vi "Measurement Logic.vi"(8 "error in":errorcluster, 9 "measurement configuration":T2={"Resource Name(s)"=[], "Number Of Records"=32, "Timeout (s)"=1.2, "Configuration File Path"="", "Delay Mode"="On", "Horizontal Position"=0.0, "Length Unit"="Percentage", "Record Length"=100.0, "Stream To File Path"=""} {"Record Length" format="%#_6ps"; "Horizontal Position" min=0.0 max=100.0 step=5.0 format="%#_6ps"; "Timeout (s)" format="%#_6p"}, 10 "measure call context in":refnum<class "Measure Call Context.lvclass">) -> (0 "error out":errorcluster, 1 "measurement results":T1={"RelativeInitialX"=[0.0], "xIncrement"=[0.0], "Wfm"=[[0.0]], "Plot Names"=[], "Actual Sample Rate"=10000000.0, "Actual Record Duration"=0.0, "Actual Record Length"=256.0} {"Actual Record Length" format="%#_6p Samples"; "Actual Record Duration" format="%#_6p Samples"; "Actual Sample Rate" format="%#_6ps"}, 2 "measure call context out":refnum<class "Measure Call Context.lvclass">)   [LabVIEW 2025, in "Ni-Scope-Multirecords.lvclass"]
doc: "Contains the core logic for executing the measurement."
uses:
  Ni-Scope-Multirecords.lvclass
  <vilib>/Plug-In SDKs/Measurements/Measure Call Context/Measure Call Context.lvclass
  Measurement Configuration.ctl
  Measurement Results.ctl
  <vilib>/Plug-In SDKs/Measurements/Measure Call Context/Reserve Sessions - NPin.vi
  <vilib>/Plug-In SDKs/Sessions/niScope/Initialize Sessions - 1Sess.vi
  <extravilib>/ChannelInstances/Event Messenger-bool/Instantiate.vi
  Ni-Scope-Multirecords.lvclass/Ni-Scope-Multirecords.ctl
  <vilib>/Plug-In SDKs/Sessions/niScope/NI Session Management niScope.lvlib
  <vilib>/Plug-In SDKs/Clients/Session Management V1/Session Reservation/Session Reservation.lvclass
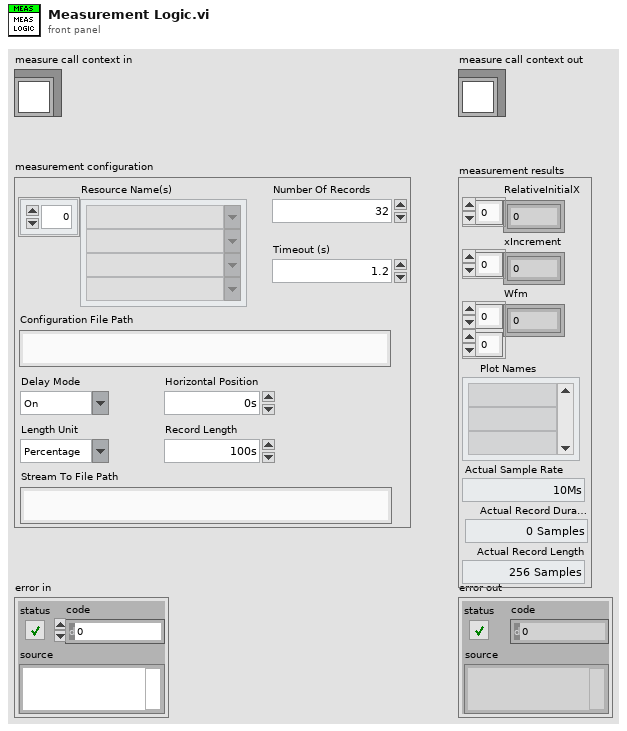
[diagram p1: front panel]
types:
  T1 = typedef "Ni-Scope-Multirecords.lvclass/Measurement Results.ctl" = cluster{"RelativeInitialX":dbl[], "xIncrement":dbl[], "Wfm":dbl[][], "Plot Names":string[], "Actual Sample Rate":dbl, "Actual Record Duration":dbl, "Actual Record Length":dbl}
  T2 = typedef "Ni-Scope-Multirecords.lvclass/Measurement Configuration.ctl" = cluster{"Resource Name(s)":string[], "Number Of Records":i32, "Timeout (s)":dbl, "Configuration File Path":string, "Delay Mode":string, "Horizontal Position":dbl, "Length Unit":string, "Record Length":dbl, "Stream To File Path":string}
  T3 = cluster{"Actual Sample Rate":dbl, "Actual Record Duration":dbl, "Actual Record Length":i32}
  T4 = typedef "Ni-Scope-Multirecords.lvclass/Recording Settings.ctl" = cluster{"Number of Records":i32, "Plot Names":string[][], "Stream To File?":bool, "TDMS Session":refnum<k34>, "Fetch Timeout":dbl, "Channels Per Record":i32}
  T5 = typedef "Event Messenger-bool.lvlib/))Channel.ctl" = refnum<queue>
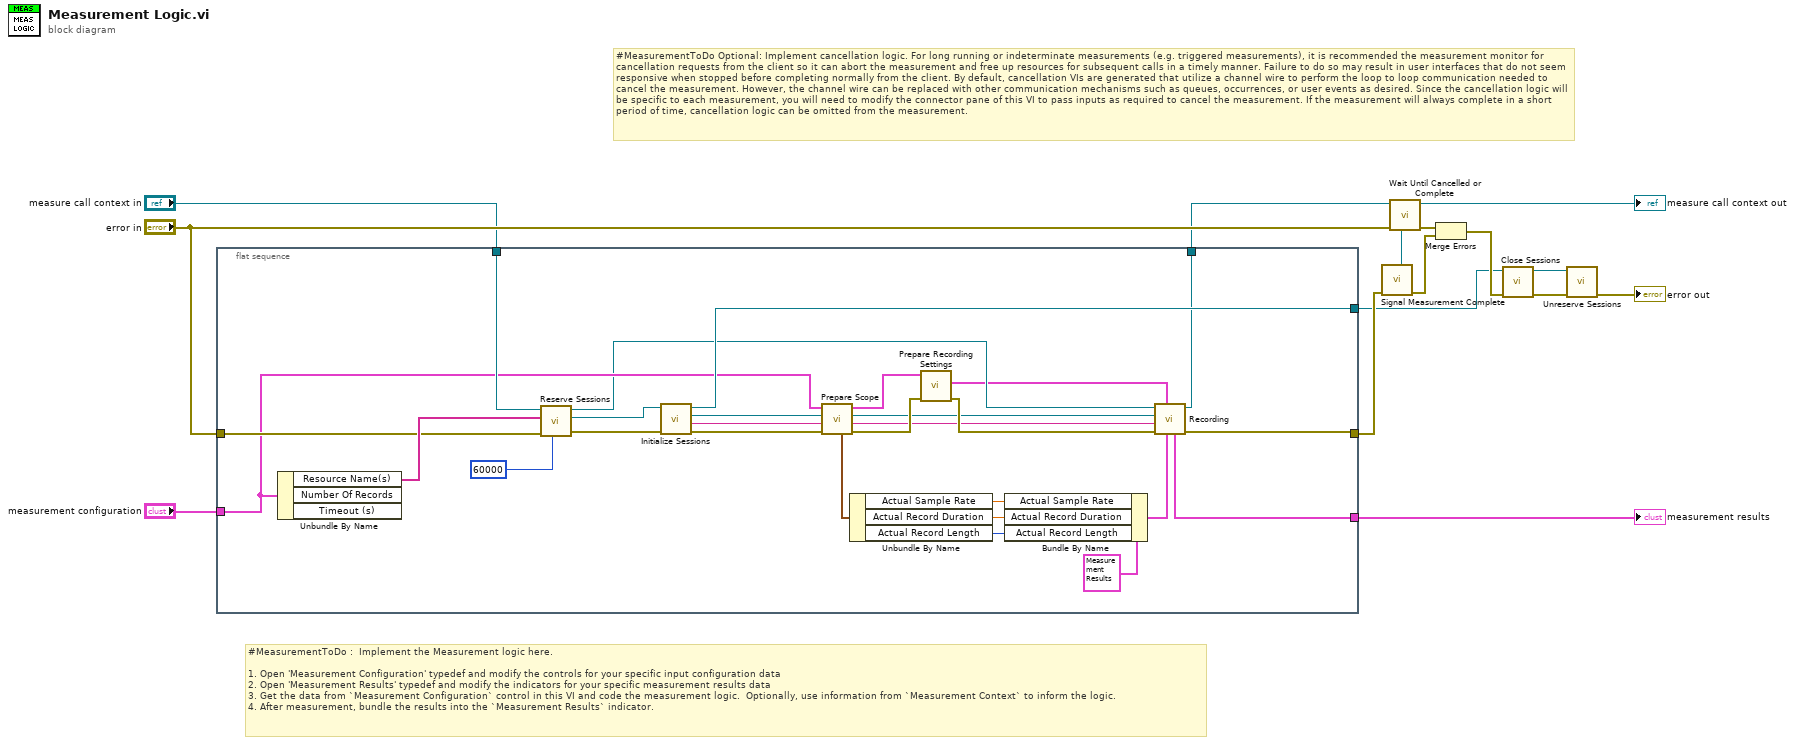
[diagram p0: block diagram]
diagram:
  # "#MeasurementToDo Optional: Implement cancellation logic. For long running or indeterminate measurements (e.g. triggered measurements), it is recommended the measurement monitor for cancellation requests from the client so it can abort the measurement and free up resources for subsequent calls in a timely manner. Failure to do so may result in user interfaces that do not seem responsive when stopped before completing normally from the client. By default, cancellation VIs are generated that utilize a channel wire to perform the loop to loop communication needed to cancel the measurement. However, the channel wire can be replaced with other communication mechanisms such as queues, occurrences, or user events as desired. Since the cancellation logic will be specific to each measurement, you will need to modify the connector pane of this VI to pass inputs as required to cancel the measurement. If the measurement will always complete in a short period of time, cancellation logic can be omitted from the measurement."
  # "#MeasurementToDo :  Implement the Measurement logic here.\n\n1. Open 'Measurement Configuration' typedef and modify the controls for your specific input configuration data\n2. Open 'Measurement Results' typedef and modify the indicators for your specific measurement results data\n3. Get the data from `Measurement Configuration` control in this VI and code the measurement logic.  Optionally, use information from `Measurement Context` to inform the logic.\n4. After measurement, bundle the results into the `Measurement Results` indicator."
  n1 = flat-sequence {
    tunnel: "measurement configuration" -> [w31]
    tunnel: [w16] -> w14
    tunnel: "error in" -> [w37]
    tunnel: [w29] -> w9
    tunnel: "measure call context in" -> [w40]
    tunnel: [w35] -> w5
    tunnel: [w25] -> w1
    frame #0 {
      n2 = Unbundle By Name(w31) -> ("Resource Name(s)"=w41:string[])  [unwired: 2 out]
      n3 = call-poly <vilib>:"Reserve Sessions.vi"("timeout (ms)"=60000, "error in"=w37, "pin or relay names"=w41, "measurement context in"=w40) -> ("error out"=w38:errorcluster, "session reservation out"=w39:refnum<class "Session Reservation.lvclass">, "measurement context out"=w26:refnum<class "Measure Call Context.lvclass">)  [unwired: 5 in]
      n4 = call-poly <vilib>:"Initialize Sessions.vi"("error in"=w38, "session reservation in"=w39) -> ("error out"=w34:errorcluster, "channel list"=w32:string, "session"=w33:refnum<k15>, "session reservation out"=w35:refnum<class "Session Reservation.lvclass">)  [unwired: 6 in]
      n5 = call "Prepare Scope.vi"("error in"=w34, "Channel List In"=w32, "Fgen Session In"=w33, "measurement configuration in"=w31) -> ("error out"=w30:errorcluster, "Channel List Out"=w18:string, "Fgen Session Out"=w19:refnum<k15>, "measurement configuration out"=w27:T2, "Actual Settings"=w20:T3)  [unwired: 3 in]
      n6 = Unbundle By Name(w20) -> ("Actual Sample Rate"=w24:dbl, "Actual Record Duration"=w23:dbl, "Actual Record Length"=w22:i32)
      n7 = call "Prepare Recording Settings.vi"("error in"=w30, "measurement configuration in"=w27) -> ("error out"=w28:errorcluster, "Recording Settings"=w21:T4)  [unwired: 7 in, 1 out]
      n8 = Bundle By Name(cluster=T1 {"RelativeInitialX"=[], "xIncrement"=[], "Wfm"=[], "Plot Names"=[], "Actual Sample Rate"=10000000.0, "Actual Record Duration"=0.0, "Actual Record Length"=256.0} ("Measurement Results"), "Actual Sample Rate"=w24, "Actual Record Duration"=w23, "Actual Record Length"=w22) -> (w17:T1)
      n9 = call "Recording.vi"("Measurement Results In"=w17, "Recording Settings"=w21, "error in"=w28, "Channel List"=w18, "FGEN Session In"=w19, "measurement context in"=w26) -> ("error out"=w29:errorcluster, "measurement context out"=w25:refnum<class "Measure Call Context.lvclass">, "Measurement Results Out"=w16:T1)  [unwired: 3 in]
    }
  }
  n10 = call "Signal Measurement Complete.vi"("error in (no error)"=w9) -> ("error out"=w12:errorcluster, "done channel"=w13:T5)  [unwired: 9 in]
  n11 = call "Wait Until Cancelled or Complete.vi"("done channel"=w13, "error in (no error)"="error in", "measure call context in"=w1) -> ("error out"=w11:errorcluster, "measure call context out"=→"measure call context out":refnum<class "Measure Call Context.lvclass">)  [unwired: 7 in]
  n12 = Merge Errors(w11, w12) -> (w6:errorcluster)
  n13 = call <vilib>:"Close Sessions.vi"("error in"=w6, "session reservation in"=w5) -> ("error out"=w8:errorcluster, "session reservation out"=w7:refnum<class "Session Reservation.lvclass">)  [unwired: 8 in]
  n14 = call <vilib>:"Unreserve Sessions.vi"("error in"=w8, "session reservation in"=w7) -> ("error out"=→"error out":errorcluster)  [unwired: 9 in]
  "measurement results" <- w14
